vi "SCREEN_1_STATE_QUEUE.vi"(7 "QUEUE ST":T2=enum."CLOSE Q", 8 "error in":errorcluster, 11 "SCREEN 1 ST":T1[](array[typedef])) -> (0 "error OUT":errorcluster, 3 "SCREEN 1":T1=enum."Cluster_Update")   [LabVIEW 2017]
uses:
  Controls/AUTO_STATE_QUEUE.ctl
  Controls/Screen1_st.ctl
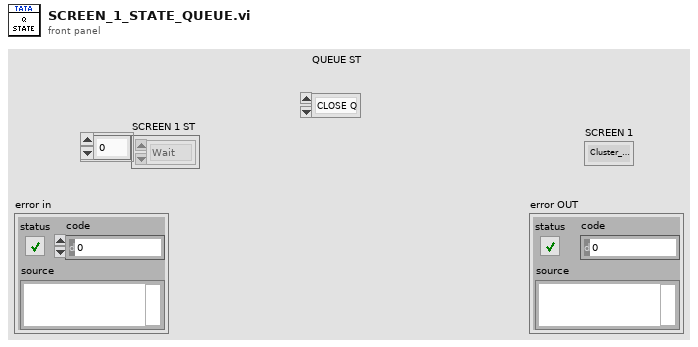
[diagram p1: front panel]
types:
  T1 = typedef "Screen1_st.ctl" = enum16{"Int", "Int2", "Wait", "Cluster_Update", "Cycle_Cmplt", "Varient_Updated", "Print_Code", "Error_Handling", "Exit"}
  T2 = typedef "AUTO_STATE_QUEUE.ctl" = enum16{"CREATE Q", "EN Q", "DE Q", "CLOSE Q"}
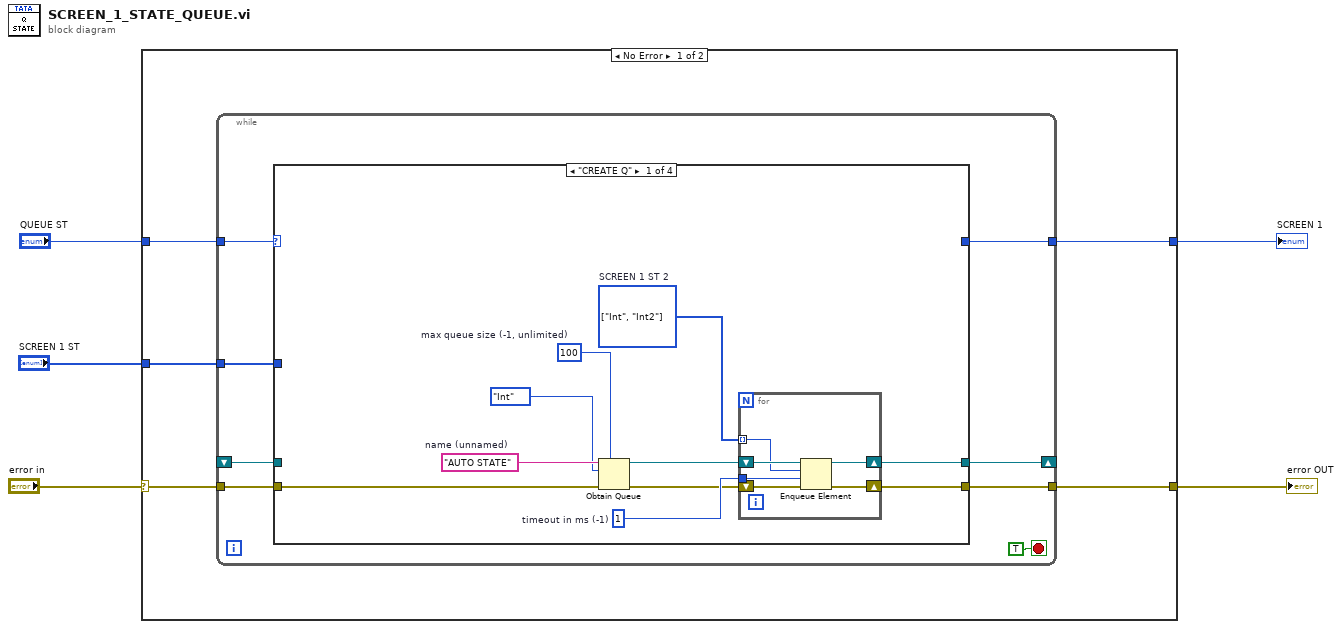
[diagram p0: block diagram]
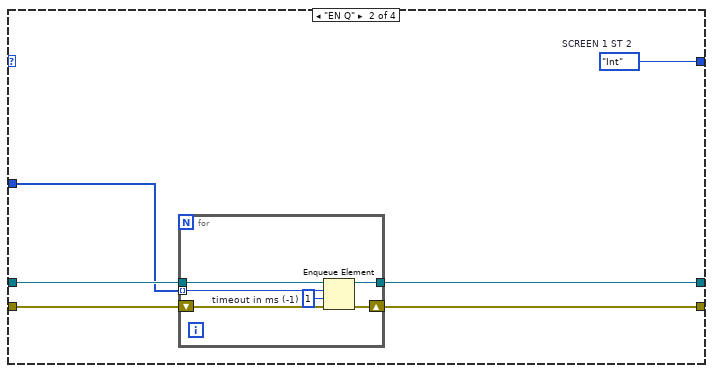
[diagram p2: hidden frame]
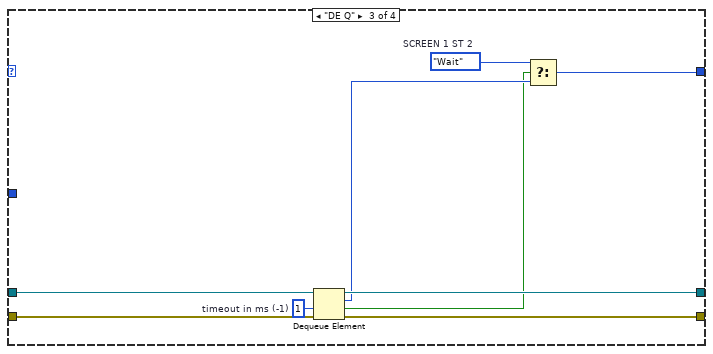
[diagram p3: hidden frame]
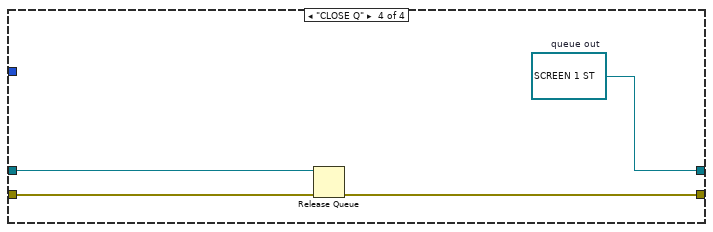
[diagram p4: hidden frame]
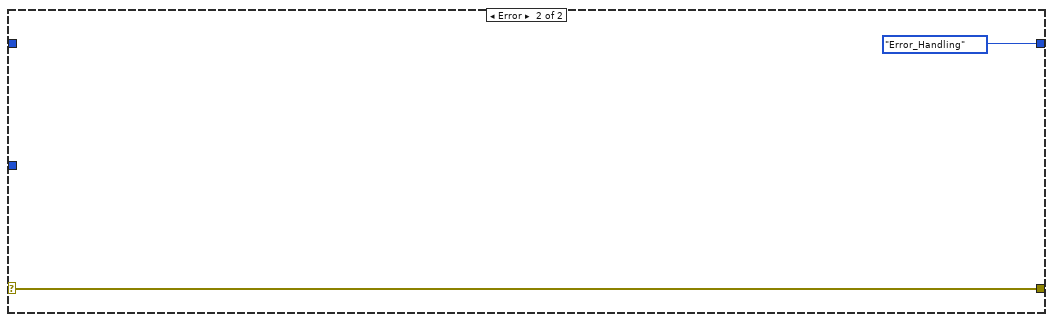
[diagram p5: hidden frame]
diagram:
  n1 = case shown="No Error" "error in" {
    selector: "error in" -> [w10 w61]
    tunnel: [w9 w61] -> w4
    tunnel: [w8 Screen1_st."Error_Handling" ("SCREEN 1 ST")] -> w1
    tunnel: "QUEUE ST" -> [w7 _]
    tunnel: "SCREEN 1 ST" -> [w6 _]
    frame No Error {
      n2 = while {
        tunnel: w10 -> [w18]
        tunnel: [w16] -> w9
        tunnel: [w11] -> w8
        tunnel: w7 -> [w15]
        shift-right: [w14] -> _
        shift-left: _ -> [w13]
        tunnel: w6 -> [w12]
        stop <- TRUE stop-if-true
        n3 = case shown="\"CREATE Q\"" w15 {
          tunnel: w18 -> [w28 w40 w55 w59]
          tunnel: [w21 w39 w54 w58] -> w16
          tunnel: [w23 w37 w52 w56] -> w14
          tunnel: w13 -> [_ w38 w53 w57]
          tunnel: w12 -> [_ w36 _ _]
          tunnel: [_ w35 w49 _] -> w11
          frame "CREATE Q" {
            w20 = T1[] [enum."Int", enum."Int2"] items=["Int", "Int2", "Wait", "Cluster_Update", "Cycle_Cmplt", "Varient_Updated", "Print_Code", "Error_Handling", "Exit"]  # SCREEN 1 ST 2
            w25 = 1  # timeout in ms (-1)
            w26 = 100  # max queue size (-1, unlimited)
            w27 = "AUTO STATE"  # name (unnamed)
            n4 = Obtain Queue(max queue size (-1, unlimited)=w26, name (unnamed)=w27, element data type=Screen1_st."Int" ("SCREEN 1 ST"), error in (no error)=w28) -> (queue out=w24:refnum<queue>, error out=w22:errorcluster)  [unwired: 1 in, 1 out]
            n5 = for {
              tunnel: w25 -> [w34]
              tunnel: w20 -> [w29] mode=indexing
              shift-right: [w32] -> w23
              shift-left: w24 -> [w33]
              shift-right: [w30] -> w21
              shift-left: w22 -> [w31]
              n6 = Enqueue Element(queue=w33, element=w29, timeout in ms (-1)=w34, error in (no error)=w31) -> (queue out=w32:refnum<queue>, error out=w30:errorcluster)  [unwired: 1 out]
            }
          }
          frame "EN Q" {
            w35 = Screen1_st."Int"  # SCREEN 1 ST 2
            n7 = for {
              tunnel: w38 -> [w44]
              tunnel: [w43] -> w37
              tunnel: w36 -> [w42] mode=indexing
              shift-right: [w45] -> w39
              shift-left: w40 -> [w46]
              w41 = 1  # timeout in ms (-1)
              n8 = Enqueue Element(queue=w44, element=w42, timeout in ms (-1)=w41, error in (no error)=w46) -> (queue out=w43:refnum<queue>, error out=w45:errorcluster)  [unwired: 1 out]
            }
          }
          frame "DE Q" {
            w47 = Screen1_st."Wait"  # SCREEN 1 ST 2
            w51 = 1  # timeout in ms (-1)
            n9 = Dequeue Element(queue=w53, timeout in ms (-1)=w51, error in (no error)=w55) -> (queue out=w52:refnum<queue>, element=w50:T1, timed out?=w48:bool, error out=w54:errorcluster)
            n10 = Select(t=w47, s=w48, f=w50) -> (s? t:f=w49:T1)
          }
          frame "CLOSE Q" {
            w56 = refnum<queue> refnum items=["Int", "Int2", "Wait", "Cluster_Update", "Cycle_Cmplt", "Varient_Updated", "Print_Code", "Error_Handling", "Exit"]  # queue out
            n11 = Release Queue(queue=w57, error in (no error)=w59) -> (error out=w58:errorcluster)  [unwired: 1 in, 2 out]
          }
        }
      }
    }
    frame Error {
    }
  }
  "error OUT" <- w4
  "SCREEN 1" <- w1
